vi "HiTechnic IRSeeker Sensor_DC all.vi"(2 "NXT":T4={"error"={"status"=FALSE, "code"=0, "source"=""}, "address"="", "NXT #"=-1, "Show Error"=TRUE, "Connection"=4} {"Connection" items=["USB", "Bluetooth", "USB then Bluetooth", "Last Connection", "Preference"]}, 3 "Port/MUX":T2 {"Port" items=["Port 1", "Port 2", "Port 3", "Port 4"]; "MUX Port" items=["No MUX", "MUX 1", "MUX 2", "MUX 3", "MUX 4"]}) -> (1 "All Info":T1, 4 "NXT":T4={"error"={"status"=FALSE, "code"=0, "source"=""}, "address"="", "NXT #"=-1, "Show Error"=TRUE, "Connection"=4} {"Connection" items=["USB", "Bluetooth", "USB then Bluetooth", "Last Connection", "Preference"]})   [LabVIEW 2009]
doc: "Reads the HiTechnic IRSeeker V2 Sensor in DC mode connected to the specified port and outputs a cluster containing the direction value as well an array of signal strengths from the five internal IR sensor elements. The direction value is in the range of 0 to 9 with 0 representing no IR detected; 1 to 9 represents a direction in a CW semi-circle around the sensor of which 5 indicates the IR source is straight ahead. In DC mode the sensor will respond to any IR source regardless if pulsating or not.\n\n<B>Inputs\nNXT </B> connects to NXT terminal of previous VI to establish the flow of the program.\n<B>Port/MUX </B> is the port used for the sensor. This is a cluster that consists of the NXT port as well as the HiTechnic Sensor Multiplexer (MUX) port. If the MUX is not used, then set this field to <B>No MUX</B>.\n\n<B>Outputs\nNXT </B> wires to NXT terminal of next VI to establish the flow of the program.\n<B>All Info </B> is a cluster containing the direction value as well as a 5 element array of signal strengths."
uses:
  <vilib>/NXT/Subs/LVHSConnector.ctl
  <vilib>/NXT/HiTechnic/subVIs/HiTechnic Port.ctl
  <vilib>/NXT/Block Support/NXT_InputPort.ctl
panel:
  # "HiTechnic IRSeeker Sensor VI\n\nThis VI reads the HiTechnic IRSeeker Sensor and \nreturns the current heading.\n\nFor more information go to www.hitechnic.com\nor email support@hitechnic.com\n(c) 2007 - 2009 HiTechnic"
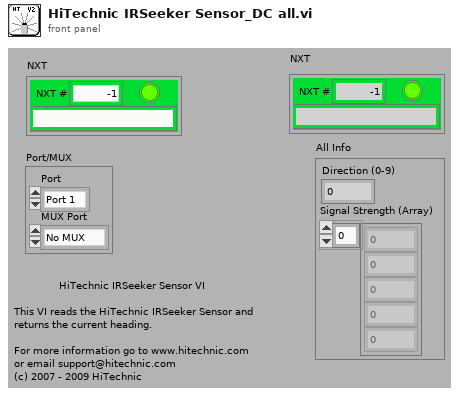
[diagram p1: front panel]
types:
  T1 = cluster{"Direction (0-9)":u8, "Signal Strength (Array)":u8[]}
  T2 = typedef "HiTechnic Port.ctl" = cluster{"Port":T3, "MUX Port":u8}
  T3 = typedef "NXT_InputPort.ctl" = u8
  T4 = typedef "LVHSConnector.ctl" = cluster{"error":errorcluster, "address":string, "NXT #":i32, "Show Error":bool, "Connection":u16}
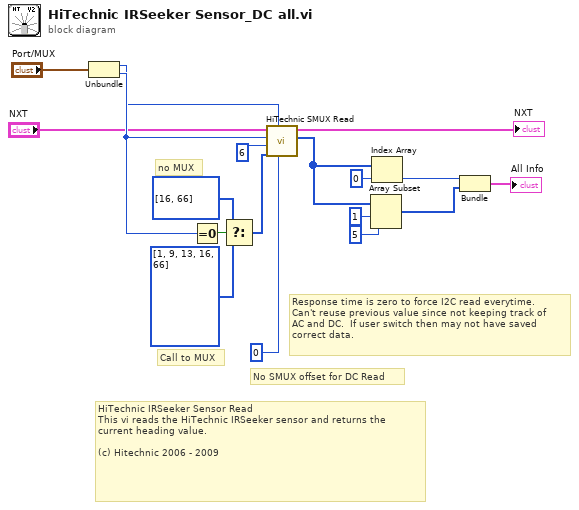
[diagram p0: block diagram]
diagram:
  # "Response time is zero to force I2C read everytime.\nCan't reuse previous value since not keeping track of\nAC and DC.  If user switch then may not have saved \ncorrect data."
  # "No SMUX offset for DC Read"
  # "no MUX"
  # "Call to MUX"
  # "HiTechnic IRSeeker Sensor Read\nThis vi reads the HiTechnic IRSeeker sensor and returns the\ncurrent heading value.  \n\n(c) Hitechnic 2006 - 2009"
  n1 = Unbundle("Port/MUX") -> ("Port"=w17:T3, "MUX Port"=w18:u8)
  n2 = Equal To 0?(x=w18) -> (x = 0?=w13:bool)
  n3 = Select(t=u8[] [16, 66] ("Buffer"), s=w13, f=u8[] [1, 9, 13, 16, 66]) -> (s? t:f=w16:u8[])
  n4 = call <vilib>:"HiTechnic SMUX Read.vi"("Offset"=u8 0, "Port"=w17, "Parameters"=w16, "Read Length"=u8 6, "MUX Port"=w18, "NXT"="NXT") -> ("Array"=w1:u8[], "NXT"=→"NXT":T4)  [unwired: 4 in]
  n5 = Array Subset(array=w1, index=1, length=5) -> (w3:u8[])
  n6 = Index Array(array=w1, index=0) -> (element=w7:u8)
  n7 = Bundle("Numeric"=w7, w3) -> (→"All Info":cluster{"Numeric":u8, u8[]})  [unwired: 1 in]
